vi "init.vi"(8 "error in (no error)":errorcluster, 11 "Actor M in":refnum<class "Actor M.lvclass">) -> (0 "error out":errorcluster, 3 "Actor M out":refnum<class "Actor M.lvclass">)   [LabVIEW 2019, in "Actor M.lvlib" / "Actor M.lvclass"]
uses:
  Actor M.lvclass
  Actor M.lvclass/Actor M.ctl
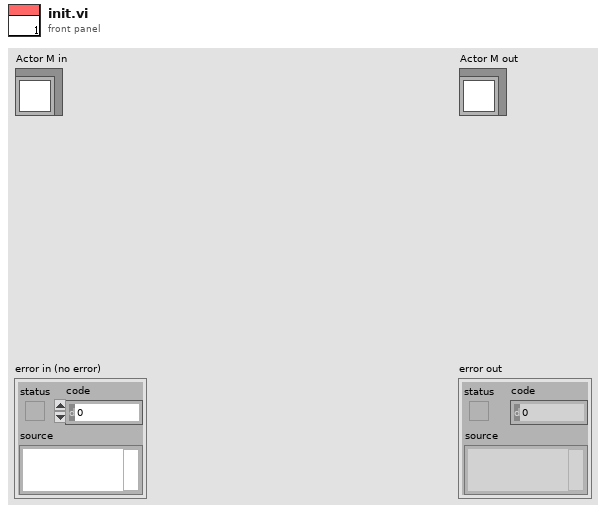
[diagram p1: front panel]
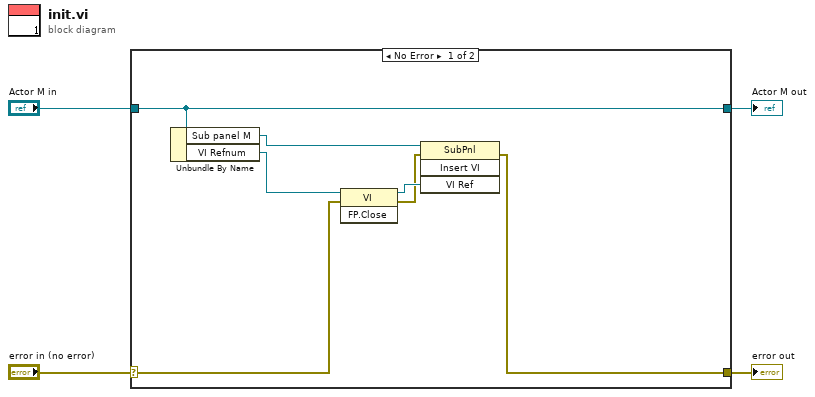
[diagram p0: block diagram]
diagram:
  n1 = case shown="No Error" "error in (no error)" {
    selector: "error in (no error)" -> [w6 w13]
    tunnel: [w5 w13] -> w3
    tunnel: [w11 w12] -> w1
    tunnel: "Actor M in" -> [w11 w12]
    frame No Error {
      n2 = Unbundle By Name(w11) -> ("Sub panel M"=w7:refnum<vi>, "VI Refnum"=w8:refnum<vi>)
      n3 = invoke class="VI" method="FP.Close"(reference=w8, error in=w6) -> (reference out=w10:refnum<vi>, error out=w9:errorcluster)  [unwired: 1 in, 1 out]
      n4 = invoke class="SubPnl" method="Insert VI"(reference=w7, error in=w9, "VI Ref"=w10) -> (error out=w5:errorcluster)  [unwired: 1 in, 3 out]
    }
    frame Error {
    }
  }
  "error out" <- w3
  "Actor M out" <- w1
